vi "Is Interface Or LabVIEW Object.vi"(10 "LabVIEW Object":refnum<class>) -> (2 "Is Interface?":bool)   [LabVIEW 2019, in "Class Integrator.lvlib"]
doc: "Checks if the provided object is an interface or LabVIEW Object."
uses:
  Class Integrator.lvlib
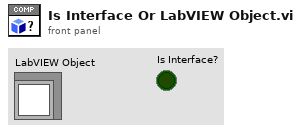
[diagram p1: front panel]
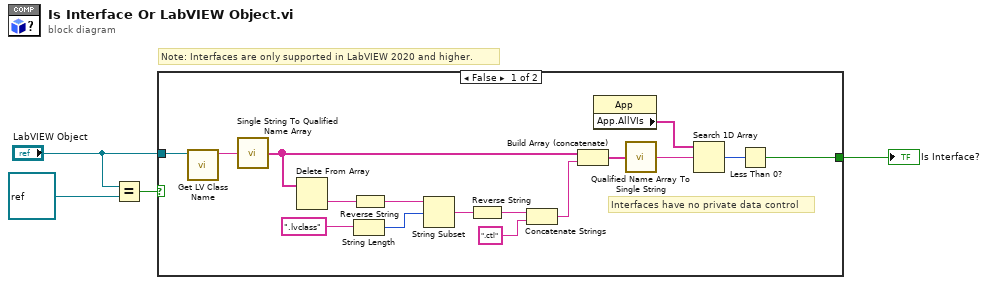
[diagram p0: block diagram]
diagram:
  # "Note: Interfaces are only supported in LabVIEW 2020 and higher."
  n1 = Equal?(x="LabVIEW Object", y=refnum<class> refnum) -> (x = y?=w3:bool)
  n2 = case shown="False" w3 {
    selector: w3 -> [_ w21]
    tunnel: "LabVIEW Object" -> [w20 _]
    tunnel: [w5 w21] -> w4
    frame False {
      # "Interfaces have no private data control"
      n3 = call <vilib>:"Get LV Class Name.vi"("object"=w20) -> ("class name"=w15:string)  [unwired: 9 in, 1 out]
      n4 = call <vilib>:"Single String To Qualified Name Array.vi"("Fully Qualified String"=w15) -> ("Fully Qualified Array"=w14:string[])
      n5 = Delete From Array(array=w14) -> (deleted portion=w13:string)  [unwired: 2 in, 1 out]
      n6 = String Length(string=".lvclass") -> (length=w18:i32)
      n7 = Reverse String(1:w13) -> (0:w17:string)
      n8 = String Subset(string=w17, offset (0)=w18) -> (substring=w16:string)  [unwired: 1 in]
      n9 = Reverse String(1:w16) -> (0:w12:string)
      n10 = Concatenate Strings(w12, ".ctl" ("string")) -> (w10:string)
      n11 = Build Array (concatenate)(w14, w10) -> (w9:string[])
      n12 = property class="App"() -> ("App.AllVIs"=w7:string[])  [unwired: 2 in, 2 out]
      n13 = call <vilib>:"Qualified Name Array To Single String.vi"("Fully Qualified Array"=w9) -> ("Fully Qualified String"=w8:string)
      n14 = Search 1D Array(1D array=w7, element=w8) -> (index of element=w6:i32)  [unwired: 1 in]
      n15 = Less Than 0?(x=w6) -> (x < 0?=w5:bool)
    }
    frame True {
    }
  }
  "Is Interface?" <- w4
